vi "zero channel.vi"(6 "Index":u32, 7 "Mean (Volts)":dbl format="%.5f") -> ()   [LabVIEW 2019]
uses:
  DAQ configuration/Sensor buffer command.ctl
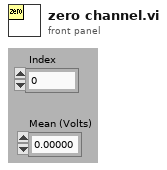
[diagram p1: front panel]
types:
  T1 = typedef "Sensor buffer command.ctl" = enum16{"read average", "read recent", "read all", "write", "set buffer size", "Read channel config", "Write channel config", "clear"}
  T2 = typedef "Channel config.ctl" = cluster{"Channel Indices":T3[], "AI Max voltage":dbl[], "Calibration matrix":T4}
  T3 = typedef "channel identifier.ctl" = u16
  T4 = typedef "calib array.ctl" = T5[]
  T5 = typedef "conversion.ctl" = cluster{"conversion matrix":sgl[][], "units":string, "name":string, "scale type":T6, "offset (volts)":dbl, "second channel":i8, "correspondence table":T7, "offset (physical units)":dbl, "pH scale":T8, "D.O.":T9, "Photometer data":T10}
  T6 = typedef "scale type.ctl" = enum16{"Volts", "Polynomial", "Correspondence Table", "pH", "Dissolved Oxygen", "Quadratic", "Photometer"}
  T7 = typedef "correspondence table.ctl" = cluster{"physical units":dbl, "volts":dbl}[]
  T8 = typedef "pH scale.ctl" = cluster{"Buffers":cluster{"Buffer":dbl, "Calibrated":bool, "V/T":dbl}[], "Temperature":dbl}
  T9 = typedef "DO scale.ctl" = cluster{"Temperature":dbl, "K":dbl, "barometric pressure":dbl}
  T10 = typedef "Photometer calibration data.ctl" = cluster{"Dark Voltage":dbl, "Blank Voltage":dbl, "Standards":cluster{"Concentration":dbl, "Voltage":dbl}[]}
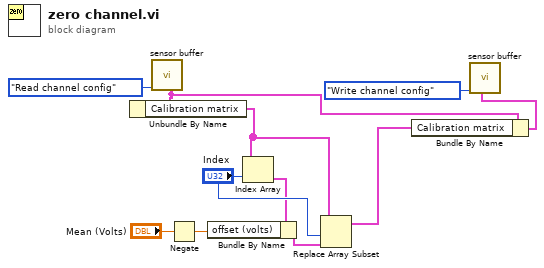
[diagram p0: block diagram]
diagram:
  n1 = call "sensor buffer.vi"("command"=Sensor_buffer_command."Read channel config") -> ("Channel Config out"=w3:T2)  [unwired: 6 in, 4 out]
  n2 = Unbundle By Name(w3) -> ("Calibration matrix"=w4:T4)
  n3 = Negate(x="Mean (Volts)") -> (-x=w7:dbl)
  n4 = Index Array(array=w4, index="Index") -> (element=w10:T5)
  n5 = Bundle By Name(cluster=w10, "offset (volts)"=w7) -> (w8:T5)
  n6 = Replace Array Subset(array=w4, new element=w8, index="Index") -> (w2:T4)
  n7 = Bundle By Name(cluster=w3, "Calibration matrix"=w2) -> (w1:T2)
  n8 = call "sensor buffer.vi"("Channel Config"=w1, "command"=Sensor_buffer_command."Write channel config") -> ()  [unwired: 5 in, 5 out]
